vi "Parallel CR read.vi"(0 "Port Base Address":u32) -> (1 "-Strobe":bool, 2 "-AutoLF":bool, 3 "-Init":bool, 4 "-Select In":bool)   [LabVIEW 2014]
doc: "Read from Control Register of Parallel Port\nThis VI determines the control register configuration of a parallel port. The four named bits may be low(F) or high(T). The Port Base Address should be the _base_ address; from there the VI gets the address of the control register itself.\nNote that this gets the actual output at the connector. You need not worry about the fact that for some bits the register is actually inverted relative to the output. This is separate from the fact that they may be 'active low' (which they all are under normal use).\nThis VI uses the National Instruments AccessHW package to access the registers under Windows XP."
uses:
  <vilib>/Platform/portaccess.llb/In Port8.vi
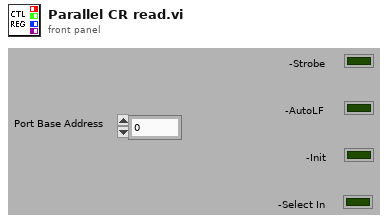
[diagram p1: front panel]
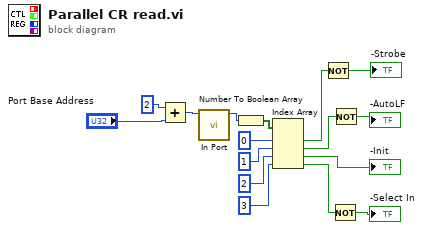
[diagram p0: block diagram]
diagram:
  n1 = Add(x=u32 2, y="Port Base Address") -> (x+y=w2:u32)
  n2 = call-poly <vilib>:"In Port.vi"("address"=w2) -> ("data read"=w1:i8)  [unwired: 7 in, 1 out]
  n3 = Number To Boolean Array(number=w1) -> (Boolean array=w14:bool[])
  n4 = Index Array(array=w14, index #1=0 ("index"), index #2=1 ("index"), index #3=2 ("index"), index #4=3 ("index")) -> (element #1=w9:bool, element #2=w8:bool, element #3=→"-Init":bool, element #4=w6:bool)
  n5 = Not(x=w9) -> (.not. x?=→"-Strobe":bool)
  n6 = Not(x=w6) -> (.not. x?=→"-Select In":bool)
  n7 = Not(x=w8) -> (.not. x?=→"-AutoLF":bool)
